vi "rs3 get frame data2.vi"(8 "error in (no error)":errorcluster, 9 "size":cluster{"width":u32, "height":u32}, 10 "stream type":u16(ring) items=["depth", "color", "inf 1", "inf 2"], 11 "device in":u64) -> (0 "error out":errorcluster, 1 "2D Color Output":u32[][](array[numeric]), 2 "2D Depth Output":u16[][](array[numeric]), 3 "device out":u64, 5 "image pointer out":u64)   [LabVIEW 2023]
doc: "With a FRAME handle as input, this will return a pointer to the actual image data. \nUse the different MEMCOPY VIs to copy the data into LabVIEW."
panel:
  # "RS3 Get Frame Data 2"
  # "(C) Intel Corp. 2017,  AGJ"
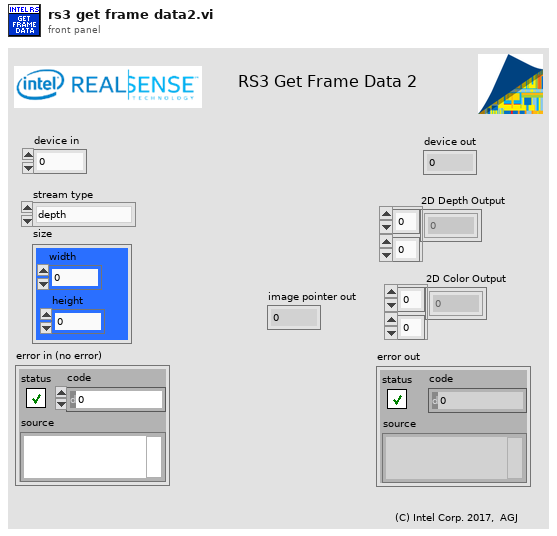
[diagram p1: front panel]
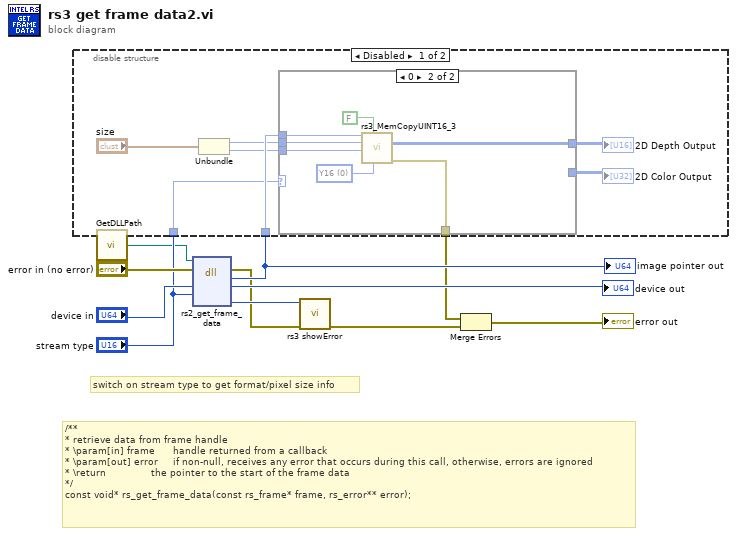
[diagram p0: block diagram]
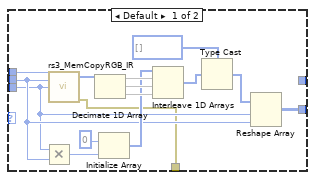
[diagram p2: hidden frame]
diagram:
  # "switch on stream type to get format/pixel size info"
  # "/**\n* retrieve data from frame handle\n* \\param[in] frame      handle returned from a callback\n* \\param[out] error     if non-null, receives any error that occurs during this call, otherwise, errors are ignored\n* \\return               the pointer to the start of the frame data\n*/\nconst void* rs_get_frame_data(const rs_frame* frame, rs_error** error);"
  n1 = call "GetDLLPath.vi"() -> ("DLL Path"=w1:path)
  n2 = dll-call lib="C:/STEAMSyndicate/RealSenseWrappers/VI Wrappers (add ons) Public/RealSense/realsense2.dll" fn="rs2_get_frame_data"(path in=w1, error in="error in (no error)", "device"="device in", "streamType"="stream type") -> (error out=w6:errorcluster, "return type"=w8:u64, "device"=→"device out":u64, "error"=w7:u64)  [unwired: 3 in, 1 out]
  "image pointer out" <- w8
  n3 = disable-structure shown="Disabled" {
    disable-tunnel: w8 -> [w19 _]
    disable-tunnel: "stream type" -> [w16 _]
    disable-tunnel: [w12 _] -> w2
    frame Disabled {
      n4 = Unbundle("size") -> ("width"=w15:u32, "height"=w14:u32)
      n5 = case shown="0" w16 {
        tunnel: w19 -> [w34 w41]
        tunnel: [_ w39] -> w17
        tunnel: w15 -> [w25 w37]
        tunnel: w14 -> [w24 w36]
        tunnel: [w28 _] -> w13
        tunnel: [w20 w35] -> w12
        frame Default {
          n6 = Multiply(x=w24, y=w25) -> (x*y=w27:u32)
          n7 = call "rs3_MemCopyRGB_IR.vi"("Zimage pointer"=w34, "RGB  X, width"=w25, "RGB Y, height"=w24) -> ("Output Array"=w33:u8[], "error out"=w20:errorcluster)  [unwired: 11 in]
          n8 = Decimate 1D Array(w33) -> (w32:u8[], w31:u8[], w30:u8[])
          n9 = Initialize Array(u8 0, w27) -> (w26:u8[])
          n10 = Interleave 1D Arrays(w26, w32, w31, w30) -> (w23:u8[])
          n11 = Type Cast(type=u32[] [], x=w23) -> (*(type *) &x=w22:u32[])
          n12 = Reshape Array(w22, w24, w25) -> (w28:u32[][])
        }
        frame 0 {
          w40 = u16 0 items=["Y16", "Y8"] ("Image format")
          n13 = call "rs3_MemCopyUINT16_3.vi"("Image format"=w40, "Transpose"=FALSE, "Height"=w36, "Width"=w37, "Zimage pointer"=w41) -> ("error out"=w35:errorcluster, "2D Array Output"=w39:u16[][])  [unwired: 5 in]
        }
      }
      "2D Depth Output" <- w17
      "2D Color Output" <- w13
    }
    frame Enabled {
    }
  }
  n14 = call "rs3 showError.vi"("error in (no error)"=w6, "error"=w7) -> ("error out"=w3:errorcluster)  [unwired: 5 in, 4 out]
  n15 = Merge Errors(w2, w3) -> (→"error out":errorcluster)
